vi "Get SMO Public API enum.vi"(8 "error in (no error)":errorcluster, 11 "Instrument in":refnum<class "Instrument.lvclass">) -> (0 "error out":errorcluster, 2 "Commands":variant, 3 "Instrument out":refnum<class "Instrument.lvclass">)   [LabVIEW 2019, in "Instrument.lvclass"]
doc: "Override this VI to return a list of commands supported by your Instrument"
uses:
  Instrument.lvclass
  Typedefs/Instrument.Commands--Enum.ctl
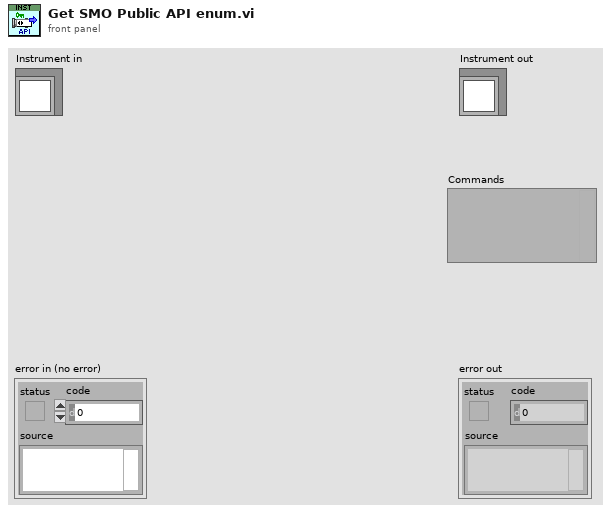
[diagram p1: front panel]
types:
  T1 = typedef "Instrument.lvclass/Instrument.Commands--Enum.ctl" = enum16{"ACK", "HELP", "setConfiguration", "setLogData", "getAll", "getAllData"}
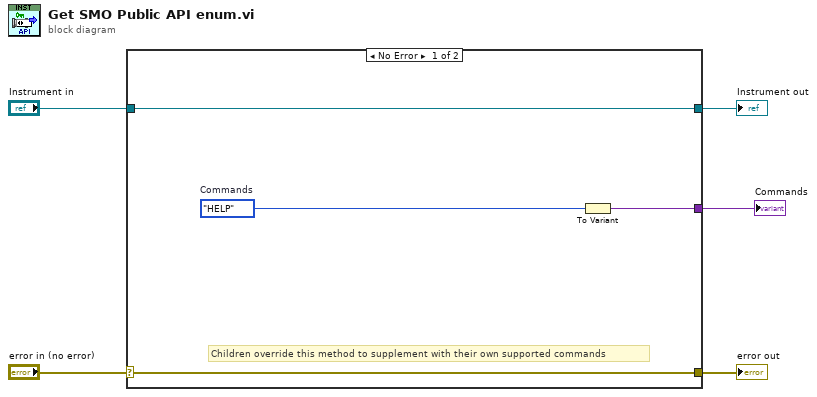
[diagram p0: block diagram]
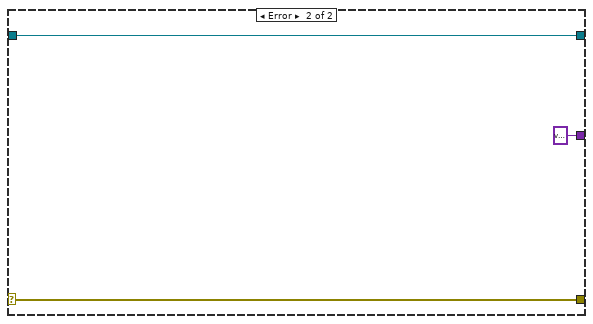
[diagram p2: hidden frame]
diagram:
  n1 = case shown="No Error" "error in (no error)" {
    selector: "error in (no error)" -> [w8 w12]
    tunnel: [w8 w12] -> w4
    tunnel: [w9 w11] -> w2
    tunnel: "Instrument in" -> [w9 w11]
    tunnel: [w6 variant ("Variant")] -> w1
    frame No Error {
      w7 = Instrument.Commands--Enum."HELP"  # Commands
      # "Children override this method to supplement with their own supported commands"
      n2 = To Variant(anything=w7) -> (Variant=w6:variant)
    }
    frame Error {
    }
  }
  "error out" <- w4
  "Instrument out" <- w2
  "Commands" <- w1
